vi "UDPsenderSimple.vi"() -> ()   [LabVIEW 2012]
panel:
  in  "Reset":bool
  in  "Send":bool
  in  "Send Command, manual entry":string
  out "Sender Error":errorcluster
  in  "End Sender Program":bool
  # "stop sender"
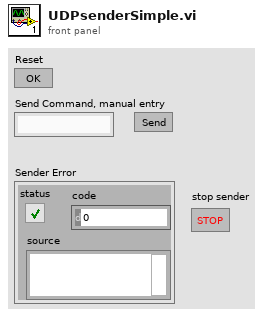
[diagram p1: front panel]
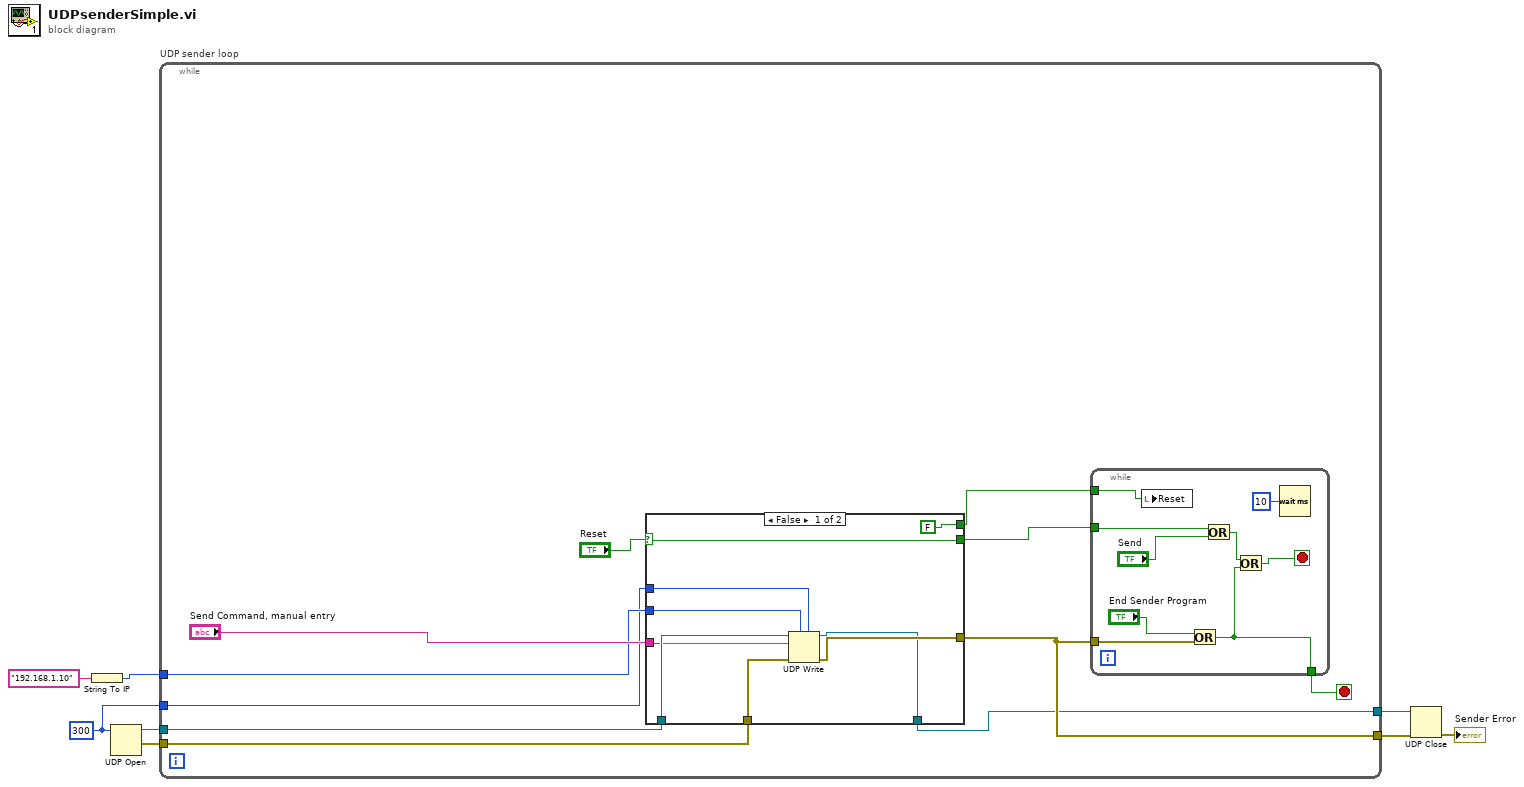
[diagram p0: block diagram]
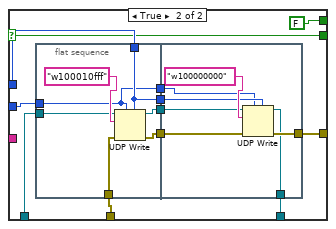
[diagram p2: hidden frame]
diagram:
  w1 = u16 300 ("port")
  n1 = String To IP(1:"192.168.1.10" ("name")) -> (0:w3:u32)
  n2 = UDP Open(11:w1) -> (port=w7:refnum<k16>, 0:w8:errorcluster)  [unwired: 4 in, 1 out]
  n3 = while "UDP sender loop" {
    tunnel: w8 -> [w16]
    tunnel: w7 -> [w14]
    tunnel: [w15] -> w6
    tunnel: w3 -> [w13]
    tunnel: [w9] -> w2
    tunnel: w1 -> [w11]
    stop <- w19 stop-if-true
    n4 = case shown="False" "Reset" {
      selector: "Reset" -> [w21 w29]
      tunnel: "Send Command, manual entry" -> [w20 _]
      tunnel: w16 -> [w27 w40]
      tunnel: [w26 w38] -> w15
      tunnel: w14 -> [w28 w35]
      tunnel: w11 -> [w23 w34]
      tunnel: w13 -> [w24 w32]
      tunnel: [FALSE ("Reset") FALSE ("Reset")] -> w10
      tunnel: [w21 w29] -> w12
      tunnel: [w25 w37] -> w9
      frame False {
        n5 = UDP Write(address=w24, port or service name=w23, connection ID=w28, data in=w20, 8:w27) -> (error out=w26:errorcluster, 3:w25:refnum<k16>)  [unwired: 1 in]
      }
      frame True {
        n6 = flat-sequence {
          tunnel: w40 -> [w46]
          tunnel: [w45] -> w39
          tunnel: [w44] -> w36
          tunnel: w35 -> [w43]
          tunnel: w34 -> [w42]
          tunnel: [w42] -> w33
          tunnel: w32 -> [w41]
          tunnel: [w41] -> w31
          tunnel: w39 -> [w53]
          tunnel: [w52] -> w38
          tunnel: [w51] -> w37
          tunnel: w36 -> [w50]
          tunnel: w33 -> [w49]
          tunnel: w31 -> [w48]
          frame #0 {
            n7 = UDP Write(address=w41, port or service name=w42, connection ID=w43, data in="w100010fff" ("F-format string"), 8:w46) -> (error out=w45:errorcluster, 3:w44:refnum<k16>)  [unwired: 1 in]
          }
          frame #1 {
            n8 = UDP Write(address=w48, port or service name=w49, connection ID=w50, data in="w100000000" ("F-format string"), 8:w53) -> (error out=w52:errorcluster, 3:w51:refnum<k16>)  [unwired: 1 in]
          }
        }
      }
    }
    n9 = while {
      tunnel: w15 -> [w61]
      tunnel: [w59] -> w19
      tunnel: w12 -> [w58]
      tunnel: w10 -> [w55]
      stop <- w62 stop-if-true
      n10 = local write "Reset"(w55) -> ()
      n11 = Or(x="End Sender Program", y=w61) -> (x .or. y?=w59:bool)
      n12 = Or(x=w58, y="Send") -> (x .or. y?=w56:bool)
      n13 = Or(x=w56, y=w59) -> (x .or. y?=w62:bool)
      n14 = Wait (ms)(milliseconds to wait=u32 10) -> ()  [unwired: 1 out]
    }
  }
  n15 = UDP Close(connection ID=w2, 8:w6) -> (error out=→"Sender Error":errorcluster)  [unwired: 1 out]
